vi "checkCOM_PortAvaliability.vi"(11 "Porta livre?":bool) -> ()   [LabVIEW 2013]
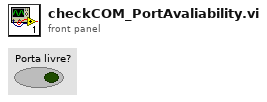
[diagram p1: front panel]
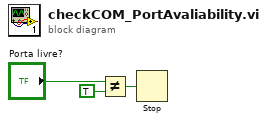
[diagram p0: block diagram]
diagram:
  n1 = Not Equal?(x="Porta livre?", y=TRUE) -> (x != y?=w3:bool)
  n2 = Stop(stop? (T)=w3) -> ()
